vi "Send ABORT.vi"(9 "Abort Request":T1={"Error URI"="wamp.error.protocol_violation", "Message"=""}, 10 "error in (no error)":errorcluster, 11 "WAMP Client in":refnum<class "WAMP Client.lvclass">) -> (2 "error out":errorcluster, 3 "WAMP Client out":refnum<class "WAMP Client.lvclass">)   [LabVIEW 2020, in "WAMP Client.lvclass"]
uses:
  <userlib>/lvwamp/WAMP Client/WAMP Client.lvclass
  <userlib>/lvwamp/WAMP Client/TypeDef/ABORT Request Data.ctl
  <userlib>/lvwamp/WAMP Client/WAMP Client.lvclass/WAMP Client.ctl
  <userlib>/lvwamp/Comm Handlers/ICommHandler/ICommHandler.lvclass
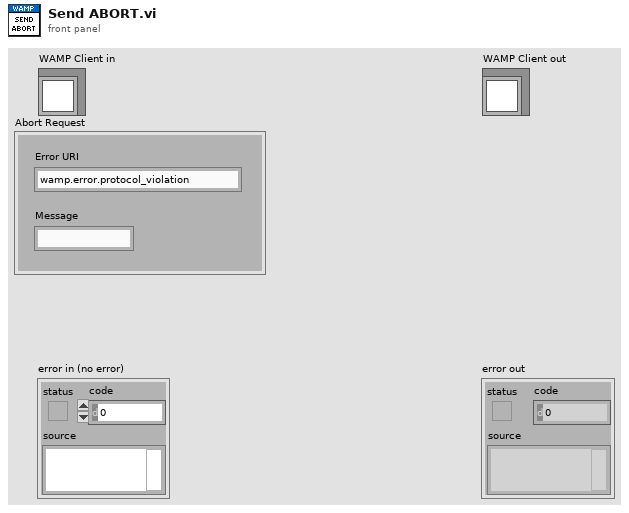
[diagram p1: front panel]
types:
  T1 = typedef "WAMP Client.lvclass/ABORT Request Data.ctl" = cluster{"Error URI":string, "Message":string}
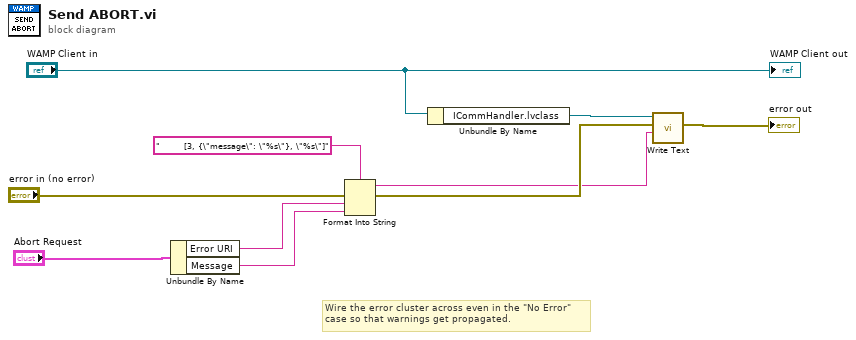
[diagram p0: block diagram]
diagram:
  # "Wire the error cluster across even in the \"No Error\"\ncase so that warnings get propagated."
  n1 = Unbundle By Name("Abort Request") -> ("Error URI"=w5:string, "Message"=w4:string)
  n2 = Format Into String(format string="        [3, {\"message\": \"%s\"}, \"%s\"]", error in="error in (no error)", w5, w4) -> (resulting string=w1:string, error out=w2:errorcluster)  [unwired: 1 in]
  n3 = Unbundle By Name("WAMP Client in") -> ("ICommHandler.lvclass"=w6:refnum<class "ICommHandler.lvclass">)
  n4 = call-dynamic "Write Text.vi"("String"=w1, "error in (no error)"=w2, "ICommHandler in"=w6) -> ("error out"=→"error out":errorcluster)  [unwired: 7 in, 1 out]
  "WAMP Client out" <- "WAMP Client in"
